vi "Range to RTD Span.vi"(8 "Floating Point Position (2)":i32=2, 9 "Scaling? (False)":bool, 10 "Type and Span":T1={"RTD Type (0 : Pt100)"=0, "Enable Span (False)"=FALSE, "Lower Span (-200.0)"=-200.0, "Upper Span (600.0)"=600.0, "Bias (0)"=0.0} {"RTD Type (0 : Pt100)" items=["Pt100", "Pt100-H", "JPt100", "JPt100-H", "Cu10GE", "Cu10LN", "Cu10WEED", "Cu10BAILEY", "Cu10a392", "Cu10a393", "Cu25", "Cu53", "Cu100", "J263B", "NI100SAMA", "NI100DIN", "NI120", "Pt25", "Pt50", "Pt200WEED", "Cu10G", "Cu50G", "Cu100G", "Pt46G", "Pt100G"]}, 11 "Temp. unit (0: C)":enum16{"C", "F"}(ring)) -> (1 "Bias":i32, 2 "Upper span":i32, 3 "Lower Span":i32)   [LabVIEW 2020, in "Yokogawa GX Series.lvlib"]
doc: "This VI gets the RTD span value from the range."
uses:
  <instrlib>/Yokogawa GX Series/Yokogawa GX Series.lvlib
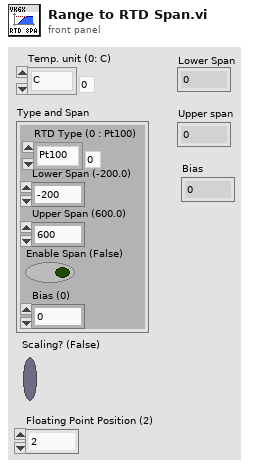
[diagram p1: front panel]
types:
  T1 = cluster{"RTD Type (0 : Pt100)":i32, "Enable Span (False)":bool, "Lower Span (-200.0)":dbl, "Upper Span (600.0)":dbl, "Bias (0)":dbl}
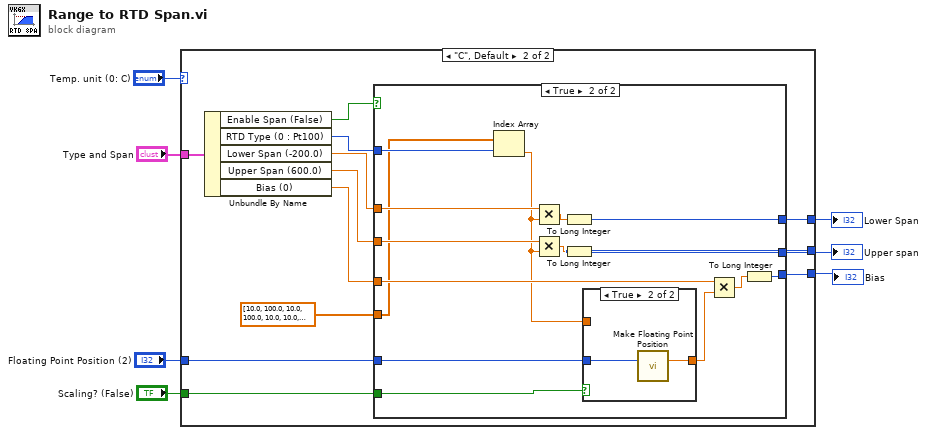
[diagram p0: block diagram]
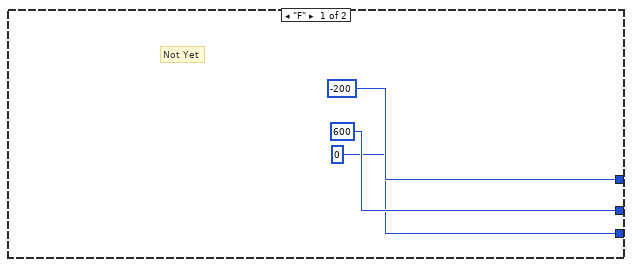
[diagram p2: hidden frame]
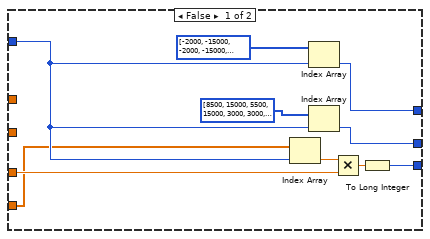
[diagram p3: hidden frame]
diagram:
  n1 = case shown="\"C\", Default" "Temp. unit (0: C)" {
    tunnel: [-200 w22] -> w5
    tunnel: [600 w21] -> w6
    tunnel: "Type and Span" -> [_ w20]
    tunnel: [0 w14] -> w3
    tunnel: "Scaling? (False)" -> [_ w13]
    tunnel: "Floating Point Position (2)" -> [_ w12]
    frame "F" {
      # "Not Yet"
    }
    frame "C", Default {
      n2 = Unbundle By Name(w20) -> ("Enable Span (False)"=w17:bool, "RTD Type (0 : Pt100)"=w16:i32, "Lower Span (-200.0)"=w19:dbl, "Upper Span (600.0)"=w18:dbl, "Bias (0)"=w15:dbl)
      n3 = case shown="True" w17 {
        tunnel: w19 -> [_ w46]
        tunnel: w18 -> [_ w45]
        tunnel: [w32 w43] -> w22
        tunnel: [w31 w42] -> w21
        tunnel: w16 -> [w30 w41]
        tunnel: w15 -> [w28 w36]
        tunnel: [w26 w40] -> w14
        tunnel: w13 -> [_ w38]
        tunnel: w12 -> [_ w37]
        tunnel: dbl[] [10.0, 100.0, 10.0, 100.0, 10.0, 10.0, 10.0, 10.0, 10.0, 10.0, 10.0, 10.0, 10.0, 10.0, 10.0, 10.0, 10.0, 10.0, 10.0, 10.0, 10.0, 10.0, 10.0, 10.0, 10.0] -> [w23 w33]
        frame False {
          n4 = Index Array(array=w23, index=w30) -> (element=w29:dbl)
          n5 = Index Array(array=i32[] [-2000, -15000, -2000, -15000, -2000, -2000, -2000, -2000, -2000, -2000, -2000, -500, -500, 0, -2000, -600, -700, -2000, -2000, -1000, -2000, -2000, -2000, -2000, -2000], index=w30) -> (element=w32:i32)
          n6 = Index Array(array=i32[] [8500, 15000, 5500, 15000, 3000, 3000, 3000, 3000, 3000, 3000, 3000, 1500, 1500, 3000, 2500, 1800, 2000, 5500, 5500, 2500, 2000, 2000, 2000, 5500, 6000], index=w30) -> (element=w31:i32)
          n7 = Multiply(x=w29, y=w28) -> (x*y=w27:dbl)
          n8 = To Long Integer(number=w27) -> (32bit integer=w26:i32)
        }
        frame True {
          n9 = Index Array(array=w33, index=w41) -> (element=w34:dbl)
          n10 = Multiply(x=w46, y=w34) -> (x*y=w47:dbl)
          n11 = Multiply(x=w45, y=w34) -> (x*y=w44:dbl)
          n12 = To Long Integer(number=w47) -> (32bit integer=w43:i32)
          n13 = To Long Integer(number=w44) -> (32bit integer=w42:i32)
          n14 = case shown="True" w38 {
            tunnel: w37 -> [_ w50]
            tunnel: [w48 w49] -> w35
            tunnel: w34 -> [w48 _]
            frame False {
            }
            frame True {
              n15 = call <instrlib>:"Make Floating Point Position.vi"("Floating Point Position (2)"=w50) -> ("Times"=w49:dbl)  [unwired: 14 in]
            }
          }
          n16 = Multiply(x=w36, y=w35) -> (x*y=w39:dbl)
          n17 = To Long Integer(number=w39) -> (32bit integer=w40:i32)
        }
      }
    }
  }
  "Upper span" <- w6
  "Lower Span" <- w5
  "Bias" <- w3
